vi "NI VeriStand - Add Input Overflow Count Channel.vi"(5 "Highlight? (F)":bool, 8 "error in (no error)":errorcluster, 10 "Channel Name":string, 11 "Parent Ref in":T1 format="%.0x") -> (0 "error out":errorcluster, 1 "Channel Ref":T1 format="%.0x", 3 "Parent Ref out":T1 format="%.0x")   [LabVIEW 2020, in "Custom Device API.lvlib"]
doc: "Adds an input overflow count channel to the device or device subsection specified by <B>Parent Ref in</B>. Input overflow count channels track the number of times the system fails to write data to an asynchronous custom device because the FIFO is full. A custom device can have only one input overflow count channel."
uses:
  <vilib>/NI VeriStand/Custom Device API/Custom Device API.lvlib
  <vilib>/NI VeriStand/Custom Device API/Custom Device Item Ref.ctl
  de0fc690-c4c9-497e-8758-36b310f7a560.vi
  <vilib>/NI VeriStand/Custom Device API/Custom Device Offline Path.vi
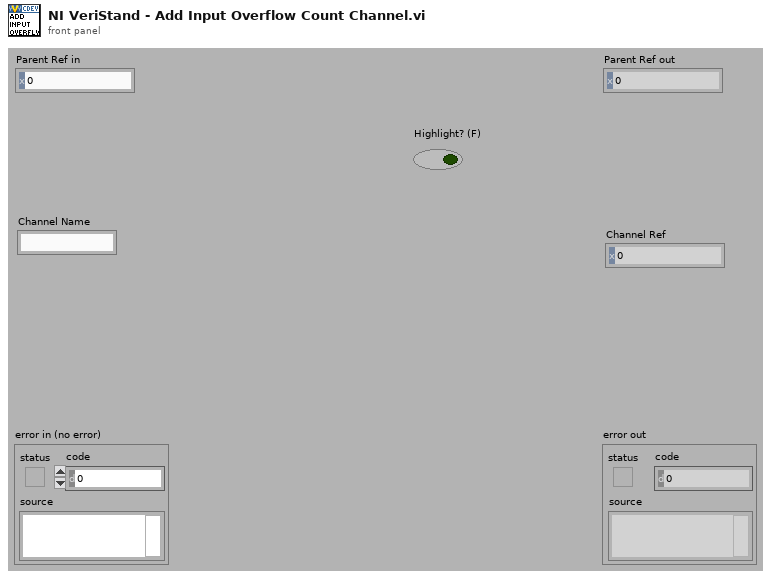
[diagram p1: front panel]
types:
  T1 = typedef "Custom Device API.lvlib/Custom Device Item Ref.ctl" = u64
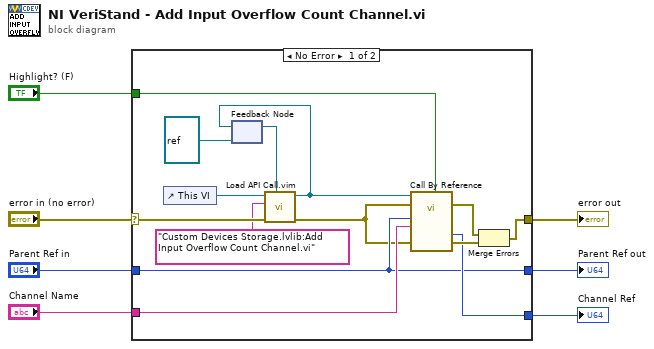
[diagram p0: block diagram]
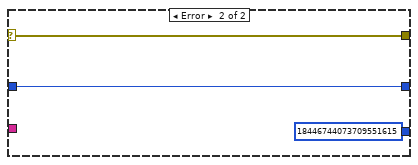
[diagram p2: hidden frame]
diagram:
  n1 = case shown="No Error" "error in (no error)" {
    selector: "error in (no error)" -> [w12 w24]
    tunnel: [w20 w24] -> w7
    tunnel: "Parent Ref in" -> [w16 w23]
    tunnel: "Channel Name" -> [w19 _]
    tunnel: "Highlight? (F)" -> [w18 _]
    tunnel: [w16 w23] -> w3
    tunnel: [w17 T1 18446744073709551615 ("Channel Ref")] -> w2
    frame No Error {
      n2 = control-ref of="This VI"() -> (w14:refnum<vi>)
      n3 = feedback #1(refnum<vi> refnum ("type specifier VI Refnum (for type only)")) -> (w15:refnum<vi>)
      n4 = call "Load API Call.vim"("VI reference in"=w15, "error in (no error)"=w12, "VI qualified name"="Custom Devices Storage.lvlib:Add Input Overflow Count Channel.vi", "Caller VI ref"=w14) -> ("error out"=w11:errorcluster, "VI reference"=w13:refnum<vi>)  [unwired: 6 in]
      n5 = feedback-in #1(w13) -> ()
      n6 = call-by-ref "?"(reference=w13, error in=w11, "Highlight? (F)"=w18, 8:"error in (no error)"=w11, "Channel Name"=w19, "Parent Ref in"=w16) -> (error out=w8:errorcluster, 0:"error out"=w21:errorcluster, "Channel Ref"=w17:T1)  [unwired: 5 in, 2 out]
      n7 = Merge Errors(w8, w21) -> (w20:errorcluster)
    }
    frame Error {
    }
  }
  "Parent Ref out" <- w3
  "error out" <- w7
  "Channel Ref" <- w2
